vi "Update Value.vi"(6 "Time":dbl, 8 "error in (no error)":errorcluster, 11 "Sequencing Control in":refnum<class "Sequencing Control.lvclass">) -> (0 "error out":errorcluster, 1 "Update":bool, 2 "Value":variant, 3 "Sequencing Control out":refnum<class "Sequencing Control.lvclass">)   [LabVIEW 2020, in "VolatusSeqGUI.lvlib" / "Sequencing Control.lvclass"]
uses:
  Sequencing Control.lvclass
  Sequencing Control.lvclass/Sequencing Control.ctl
  Loop Async.vi
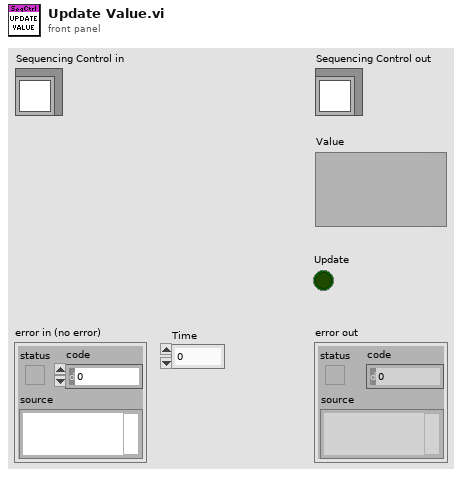
[diagram p1: front panel]
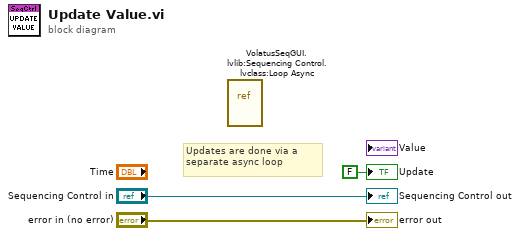
[diagram p0: block diagram]
diagram:
  # "Updates are done via a separate async loop"
  n1 = vi-ref "VolatusSeqGUI.lvlib:Sequencing Control.lvclass:Loop Async.vi"() -> ()  [unwired: 1 out]
  "error out" <- "error in (no error)"
  "Sequencing Control out" <- "Sequencing Control in"
  "Update" <- FALSE ("Update")
